vi "calculateBalance.vi"(8 "error in (no error)":errorcluster, 10 "WhichMonth":refnum<class "WhichMonth.lvclass">, 11 "Database in":refnum<class "Account History.lvclass">) -> (0 "error out":errorcluster, 2 "Month Balance":dbl, 3 "Database out":refnum<class "Account History.lvclass">)   [LabVIEW 2018, in "Account History.lvclass"]
uses:
  Account History.lvclass
  WhichMonth/WhichMonth.lvclass
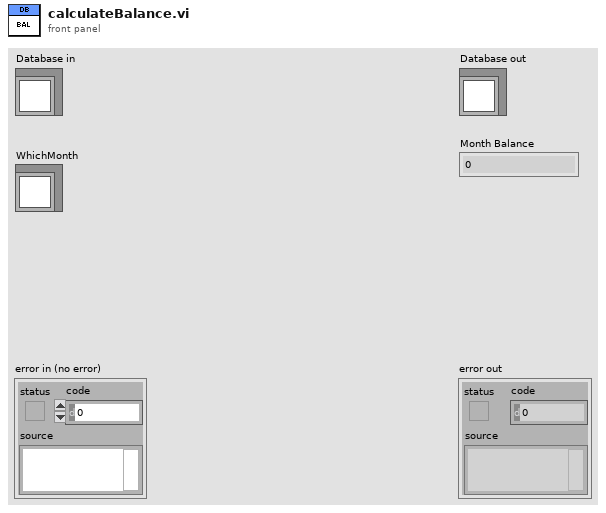
[diagram p1: front panel]
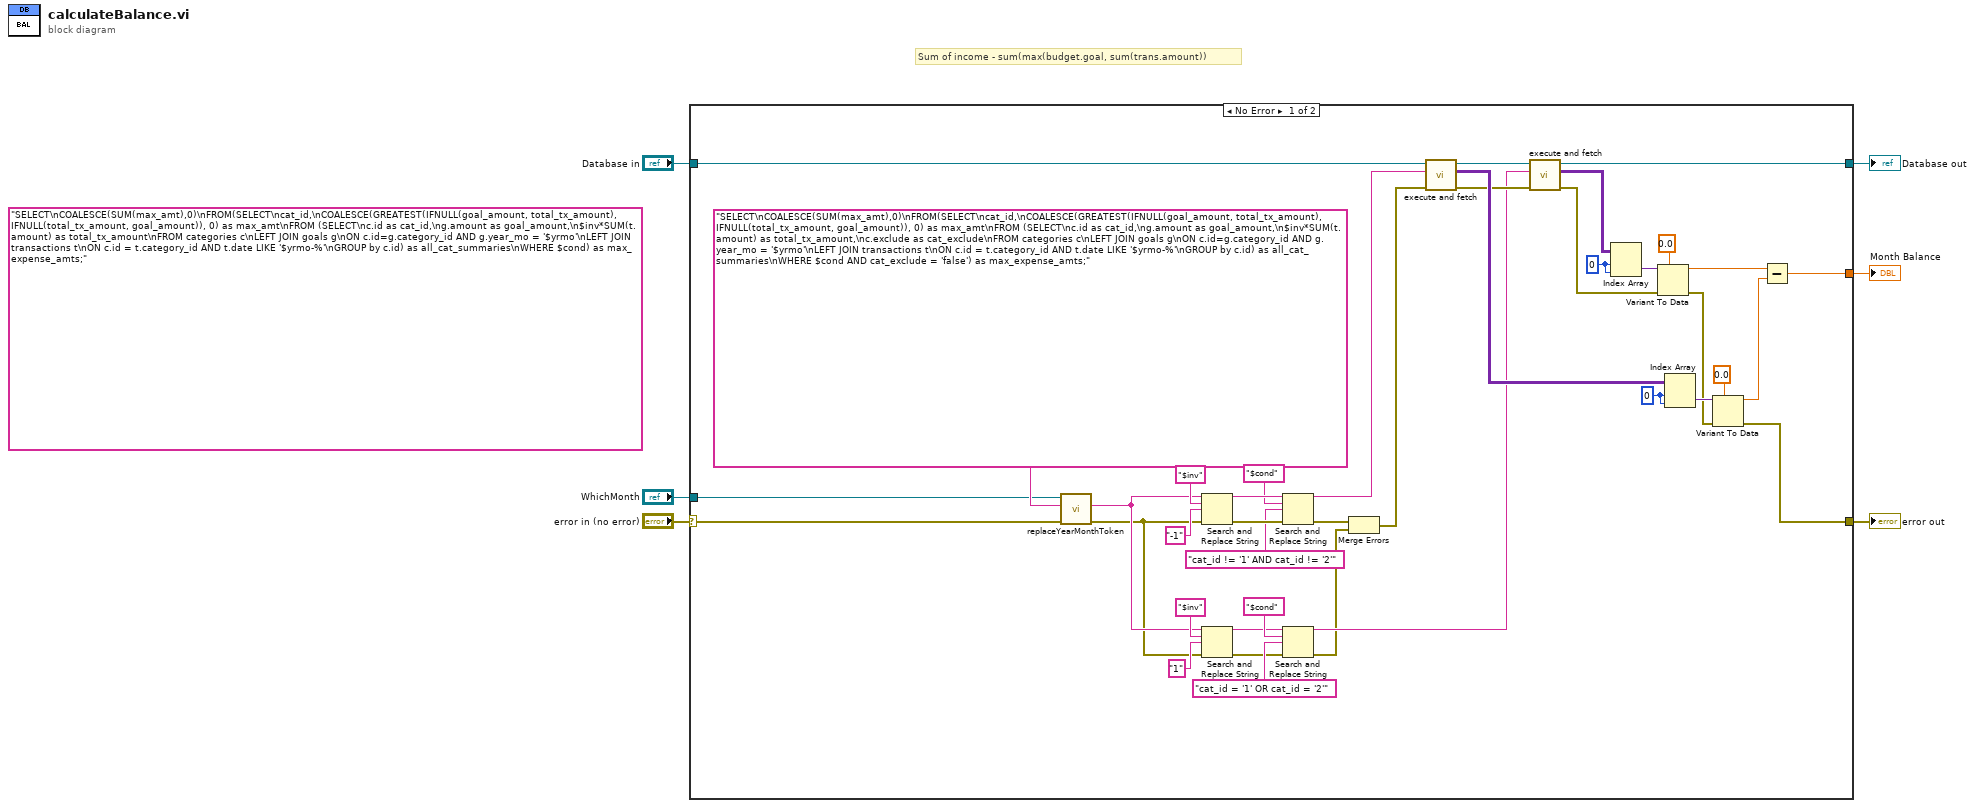
[diagram p0: block diagram]
diagram:
  (unwired) "SELECT\nCOALESCE(SUM(max_amt),0)\nFROM(SELECT\ncat_id,\nCOALESCE(GREATEST(IFNULL(goal_amount, total_tx_amount), IFNULL(total_tx_amount, goal_amount)), 0) as max_amt\nFROM (SELECT\nc.id as cat_id,\ng.amount as goal_amount,\n$inv*SUM(t.amount) as total_tx_amount\nFROM categories c\nLEFT JOIN goals g\nON c.id=g.category_id AND g.year_mo = '$yrmo'\nLEFT JOIN transactions t\nON c.id = t.category_id AND t.date LIKE '$yrmo-%'\nGROUP by c.id) as all_cat_summaries\nWHERE $cond) as max_expense_amts;"
  # "Sum of income - sum(max(budget.goal, sum(trans.amount))"
  n1 = case shown="No Error" "error in (no error)" {
    selector: "error in (no error)" -> [w12 w48]
    tunnel: [w41 w48] -> w5
    tunnel: [w20 w47] -> w3
    tunnel: "Database in" -> [w46 w47]
    tunnel: "WhichMonth" -> [w13 _]
    tunnel: [w7 _] -> w1
    frame No Error {
      w22 = 0 ("index (row)")
      w44 = 0 ("index (row)")
      n2 = call "replaceYearMonthToken.vi"("error in (no error)"=w12, "Query In"="SELECT\nCOALESCE(SUM(max_amt),0)\nFROM(SELECT\ncat_id,\nCOALESCE(GREATEST(IFNULL(goal_amount, total_tx_amount), IFNULL(total_tx_amount, goal_amount)), 0) as max_amt\nFROM (SELECT\nc.id as cat_id,\ng.amount as goal_amount,\n$inv*SUM(t.amount) as total_tx_amount,\nc.exclude as cat_exclude\nFROM categories c\nLEFT JOIN goals g\nON c.id=g.category_id AND g.year_mo = '$yrmo'\nLEFT JOIN transactions t\nON c.id = t.category_id AND t.date LIKE '$yrmo-%'\nGROUP by c.id) as all_cat_summaries\nWHERE $cond AND cat_exclude = 'false') as max_expense_amts;", "WhichMonth in"=w13) -> ("error out"=w10:errorcluster, "Query Out"=w11:string)  [unwired: 6 in, 1 out]
      n3 = Search and Replace String(input string=w11, search string="$inv", replace string="-1" ("replace string (\"\")"), error in=w10) -> (result string=w38:string, error out=w37:errorcluster)  [unwired: 4 in, 2 out]
      n4 = Search and Replace String(input string=w11, search string="$inv", replace string="1" ("replace string (\"\")"), error in=w10) -> (result string=w30:string, error out=w31:errorcluster)  [unwired: 4 in, 2 out]
      n5 = Search and Replace String(input string=w38, search string="$cond", replace string="cat_id != '1' AND cat_id != '2'" ("replace string (\"\")"), error in=w37) -> (result string=w34:string, error out=w17:errorcluster)  [unwired: 4 in, 2 out]
      n6 = Search and Replace String(input string=w30, search string="$cond", replace string="cat_id = '1' OR cat_id = '2'" ("replace string (\"\")"), error in=w31) -> (result string=w25:string, error out=w16:errorcluster)  [unwired: 4 in, 2 out]
      n7 = Merge Errors(w17, w16) -> (w15:errorcluster)
      n8 = call "execute and fetch.vi"("error in (no error)"=w15, "SQL query"=w34, "Database in"=w46) -> ("error out"=w26:errorcluster, "recordset data"=w45:variant[][], "Database out"=w27:refnum<class "Account History.lvclass">)  [unwired: 5 in, 1 out]
      n9 = call "execute and fetch.vi"("error in (no error)"=w26, "SQL query"=w25, "Database in"=w27) -> ("error out"=w19:errorcluster, "recordset data"=w21:variant[][], "Database out"=w20:refnum<class "Account History.lvclass">)  [unwired: 5 in, 1 out]
      n10 = Index Array(array=w21, index (row)=w22, index (col)=w22) -> (element=w23:variant)
      n11 = Variant To Data(error in=w19, type=0.0, Variant=w23) -> (data=w9:dbl, error out=w18:errorcluster)
      n12 = Index Array(array=w45, index (row)=w44, index (col)=w44) -> (element=w43:variant)
      n13 = Variant To Data(error in=w18, type=0.0, Variant=w43) -> (data=w8:dbl, error out=w41:errorcluster)
      n14 = Subtract(x=w9, y=w8) -> (x-y=w7:dbl)
    }
    frame Error {
    }
  }
  "error out" <- w5
  "Database out" <- w3
  "Month Balance" <- w1
